vi "Exercise4.vi"() -> ()   [LabVIEW 2019]
panel:
  out "Gauge":dbl(knob) scale=0.0..20.0
  in  "Down Button":bool
  in  "Up Button":bool
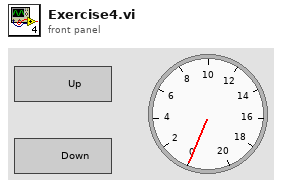
[diagram p1: front panel]
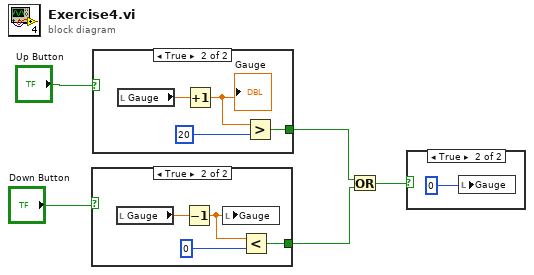
[diagram p0: block diagram]
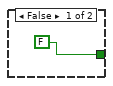
[diagram p3: hidden frame]
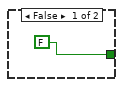
[diagram p4: hidden frame]
diagram:
  n1 = case shown="True" "Down Button" {
    tunnel: [FALSE w7] -> w2
    frame False {
    }
    frame True {
      n2 = local read "Gauge"() -> (w10:dbl)
      n3 = Decrement(x=w10) -> (x-1=w8:dbl)
      n4 = local write "Gauge"(w8) -> ()
      n5 = Less?(x=w8, y=0) -> (x < y?=w7:bool)
    }
  }
  n6 = case shown="True" "Up Button" {
    tunnel: [FALSE w12] -> w3
    frame False {
    }
    frame True {
      n7 = local read "Gauge"() -> (w15:dbl)
      n8 = Increment(x=w15) -> (x+1=w13:dbl)
      "Gauge" <- w13
      n9 = Greater?(x=w13, y=20) -> (0:w12:bool)
    }
  }
  n10 = Or(x=w3, y=w2) -> (x .or. y?=w1:bool)
  n11 = case shown="True" w1 {
    frame False {
    }
    frame True {
      n12 = local write "Gauge"(0) -> ()
    }
  }
